vi "Read Event - New Song.vi"(8 "error in (no error)":errorcluster, 11 "SongPlayerActor in":refnum<class "SongPlayerActor.lvclass">) -> (0 "error out":errorcluster, 2 "Event - New Song":refnum<user-event>, 3 "SongPlayerActor out":refnum<class "SongPlayerActor.lvclass">)   [LabVIEW 2015, in "SongPlayerActor.lvlib" / "SongPlayerActor.lvclass"]
uses:
  SongPlayerActor.lvclass
  file/MusicElement/Song/Song.lvclass
  SongPlayerActor.lvclass/SongPlayerActor.ctl
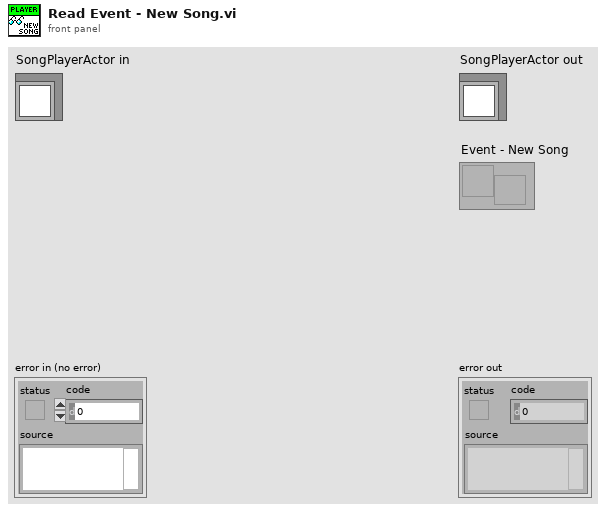
[diagram p1: front panel]
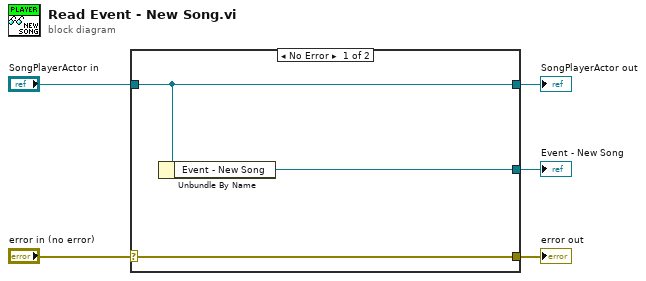
[diagram p0: block diagram]
diagram:
  n1 = case shown="No Error" "error in (no error)" {
    selector: "error in (no error)" -> [w8 w9]
    tunnel: [w8 w9] -> w4
    tunnel: [w7 w10] -> w2
    tunnel: "SongPlayerActor in" -> [w7 w10]
    tunnel: [w6 _] -> w1
    frame No Error {
      n2 = Unbundle By Name(w7) -> ("Event - New Song"=w6:refnum<user-event>)
    }
    frame Error {
    }
  }
  "error out" <- w4
  "SongPlayerActor out" <- w2
  "Event - New Song" <- w1
